vi "手動.vi"() -> ()   [LabVIEW 2015]
panel:
  out "Ready":bool
  out "Tab 機構部件":T1(tab)
  in  "Recipe Ring":u8(ring) items=["TraySize 3x7_Position.ini", "TraySize 5x8"]
  in  "機構部件":T1(ring)
  in  "Exit":bool
  # "手動"
  # "單部動作"
  # "汽缸作動"
  # "目標位置移動"
  # "單部動作"
  # "汽缸作動"
  # "目標位置移動"
  # "單部動作"
  # "汽缸作動"
  # "目標位置移動"
  # "單部動作"
  # "汽缸作動"
  # "單部動作"
  # "汽缸作動"
  # "目標位置移動"
  # "單部動作"
  # "汽缸作動"
  # "目標位置移動"
  # "單部動作"
  # "汽缸作動"
  # "單部動作"
  # "汽缸作動"
  # "單部動作"
  # "汽缸作動"
  # "單部動作"
  # "汽缸作動"
  # "目標位置移動"
  # "單部動作"
  # "汽缸作動"
  # "目標位置移動"
  # "單部動作"
  # "汽缸作動"
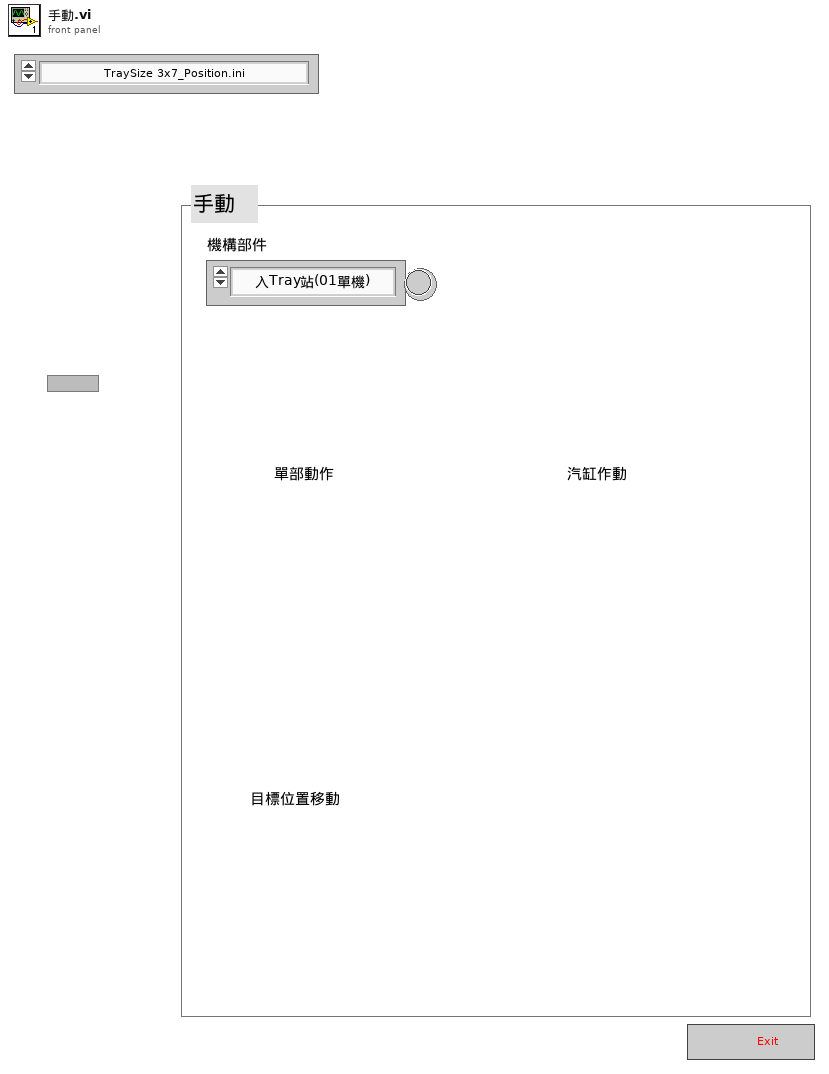
[diagram p1: front panel]
types:
  T1 = enum32{"入Tray站(01單機)", "入料站(02單機)", "對位站(02單機)", "撕膜站(03單機)", "Ag站(04單機)", "UV站(05單機)", "對折站(06單機)", "固化站(07單機)", "噴碼站(08單機)", "出料站(09單機)", "出Tray站(10單機)", "Index站"}
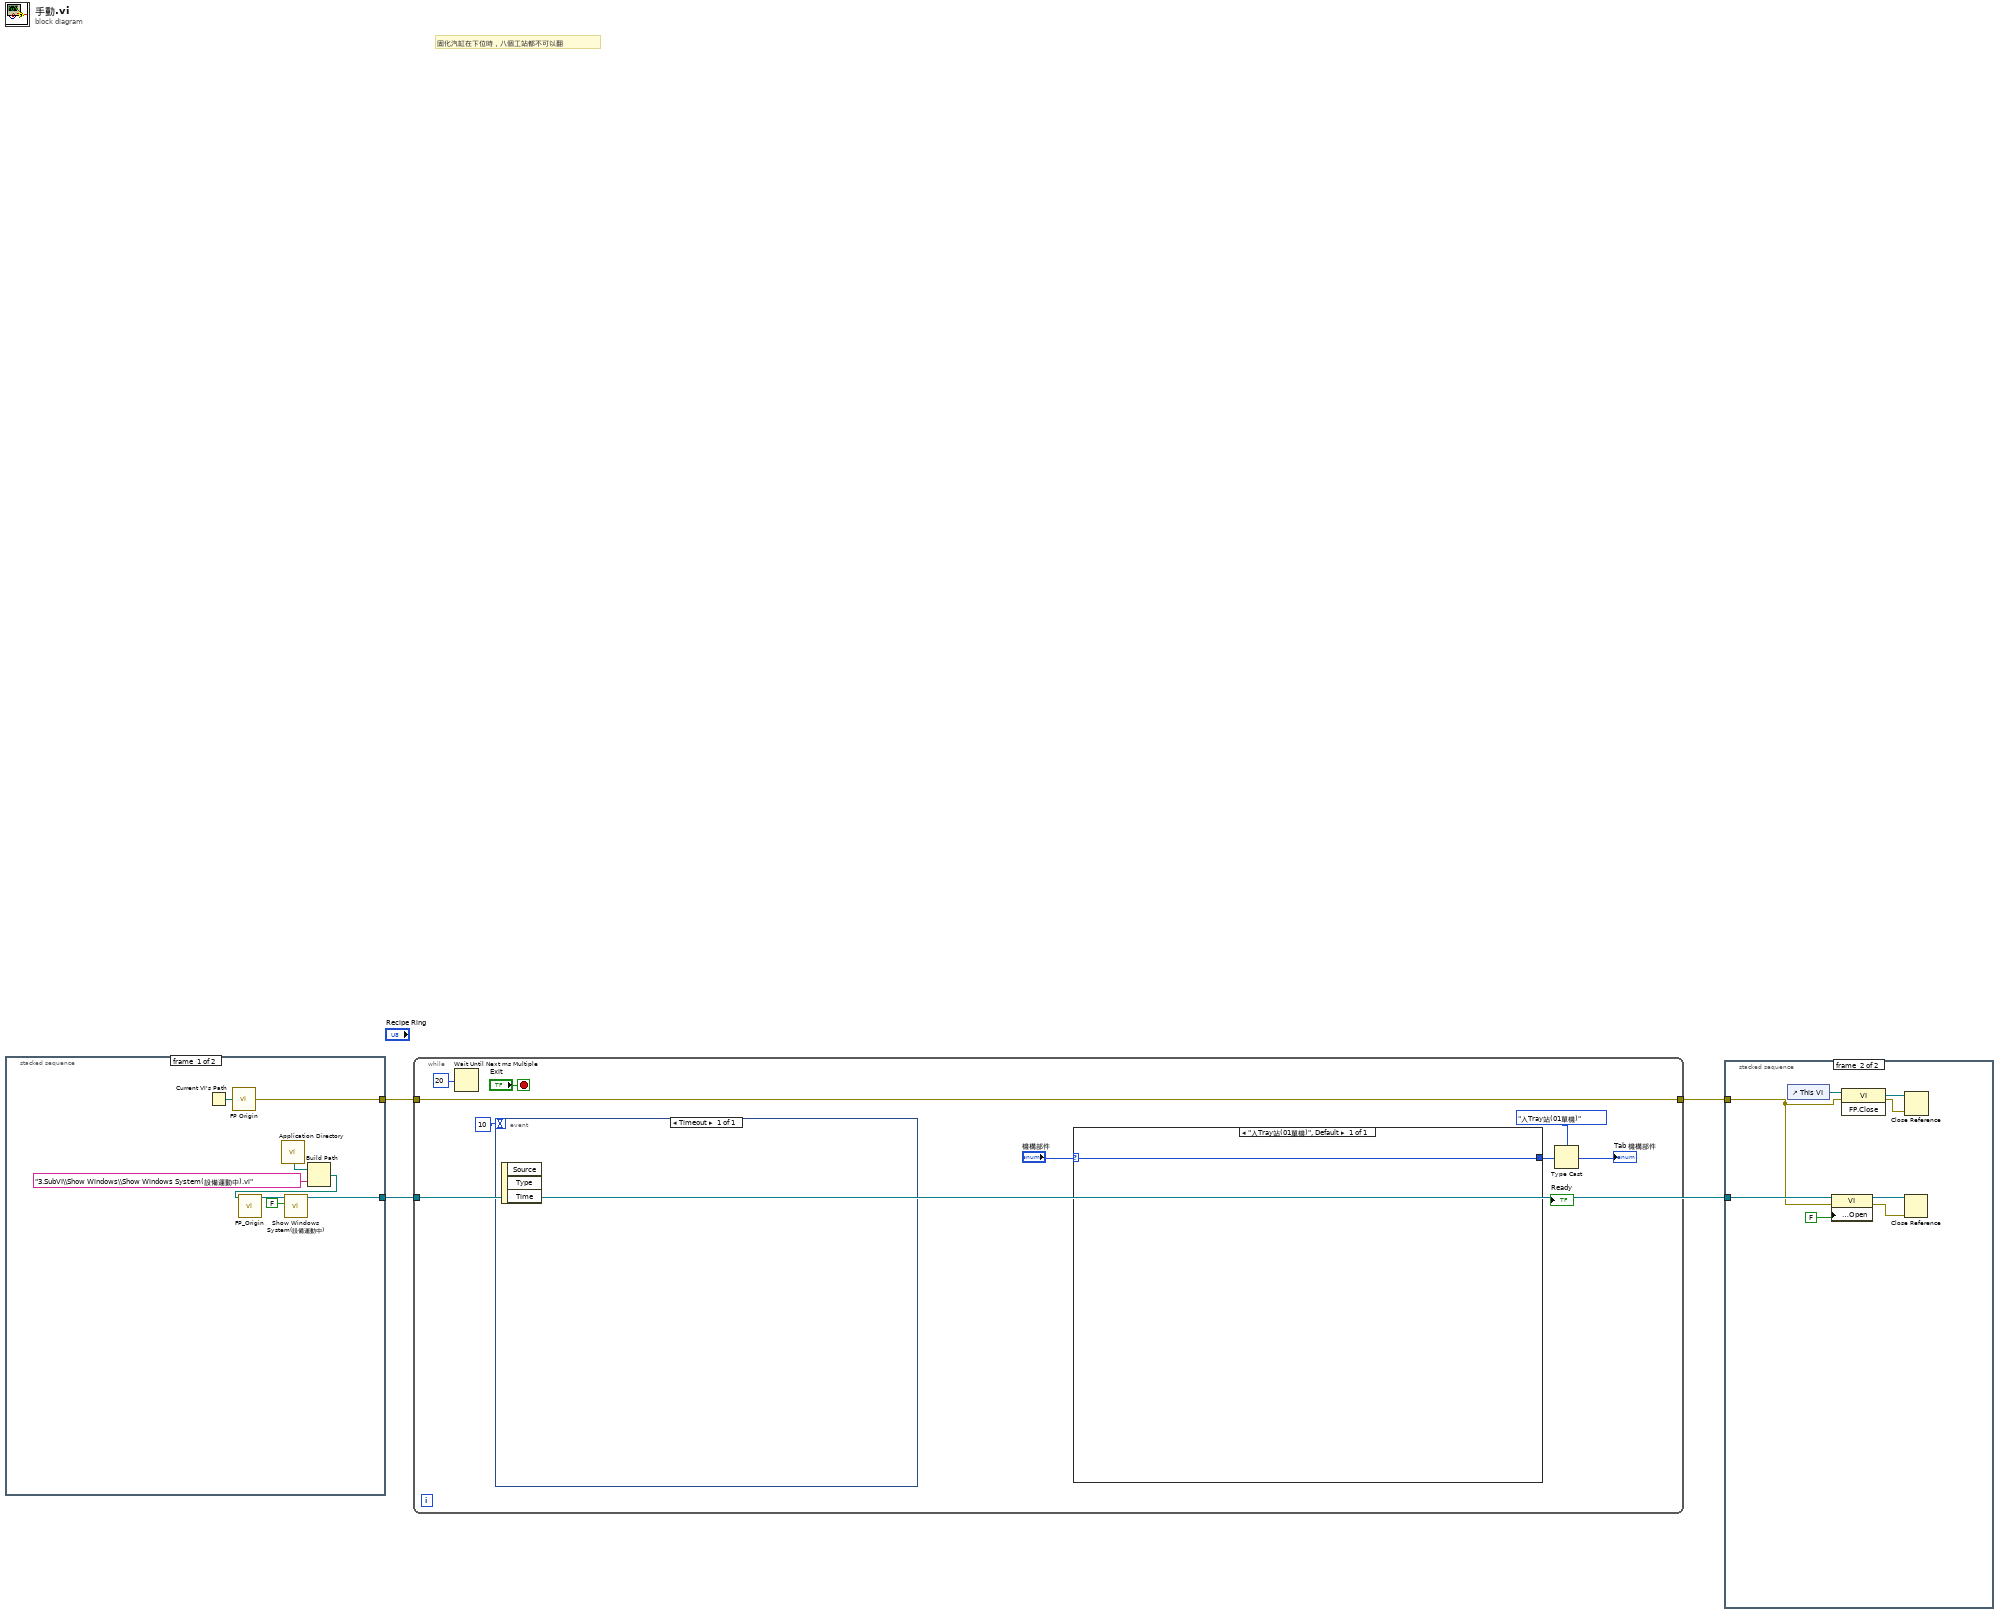
[diagram p0: block diagram]
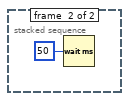
[diagram p3: hidden frame]
diagram:
  # "固化汽缸在下位時，八個工站都不可以翻"
  n1 = stacked-sequence {
    tunnel: [w10 _] -> w1
    tunnel: [w4 _] -> w2
    frame #0 {
      n2 = Current VI's Path() -> (path=w11:path)
      n3 = call "FP Origin.vi"("vi path"=w11) -> ("error out"=w10:errorcluster)
      n4 = call <vilib>:"Application Directory.vi"() -> ("Application Directory"=w9:path)
      n5 = Build Path(base path=w9, name or relative path="3.SubVI\\Show Windows\\Show Windows System(設備運動中).vi") -> (appended path=w5:path)
      n6 = call "FP_Origin.vi"("VI.Path"=w5) -> ("VI Reference"=w7:refnum<vi>)  [unwired: 9 in, 1 out]
      n7 = call "Show Windows System(設備運動中).vi"("Show"=FALSE, "vi reference in"=w7) -> ("vi reference out"=w4:refnum<vi>)  [unwired: 8 in, 1 out]
    }
    frame #1 {
      n8 = Wait (ms)(milliseconds to wait=u32 50) -> ()  [unwired: 1 out]
    }
  }
  n9 = while {
    tunnel: w1 -> [w18]
    tunnel: [w18] -> w3
    tunnel: w2 -> [_]
    stop <- "Exit" stop-if-true
    n10 = Wait Until Next ms Multiple(millisecond multiple=u32 20) -> ()  [unwired: 1 out]
    n11 = event shown="[0] Timeout" {
      selector: _ -> [_]
      dyn-events: _ -> [_]
      timeout: 10 -> [_]
      event Timeout {
        n12 = event-data() -> ()  [unwired: 1 in, 3 out]
      }
    }
    n13 = case shown="\"入Tray站(01單機)\", Default" "機構部件" {
      selector: "機構部件" -> [w21]
      tunnel: [w21] -> w16
      frame "入Tray站(01單機)", Default {
      }
    }
    n14 = Type Cast(type=T1."入Tray站(01單機)" ("Tab 機構部件"), x=w16) -> (*(type *) &x=→"Tab 機構部件":T1)
  }
  n15 = stacked-sequence {
    tunnel: w3 -> [_ w22]
    tunnel: w2 -> [_ w23]
    frame #0 {
    }
    frame #1 {
      n16 = control-ref of="This VI"() -> (w29:refnum<vi>)
      n17 = property class="VI"(reference=w23, error in=w22, "Front Panel.Open"=FALSE ("Front Panel Window:Open")) -> (reference out=w26:refnum<vi>, error out=w24:errorcluster)
      n18 = invoke class="VI" method="FP.Close"(reference=w29, error in=w22) -> (reference out=w28:refnum<vi>, error out=w27:errorcluster)  [unwired: 1 in, 1 out]
      n19 = Close Reference(reference=w26, error in (no error)=w24) -> ()  [unwired: 1 out]
      n20 = Close Reference(reference=w28, error in (no error)=w27) -> ()  [unwired: 1 out]
    }
  }
